vi "Log Data to File.vi"(8 "error in":errorcluster, 10 "Log Data":string[](array[string])) -> (0 "error out":errorcluster)   [LabVIEW 2019]
doc: "This VI writes data to Spreadsheet. Data is logged into Application Directory in CSV format."
uses:
  <vilib>/Utility/file.llb/Write Delimited Spreadsheet (string).vi
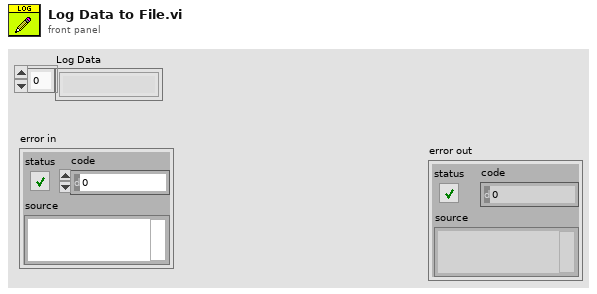
[diagram p1: front panel]
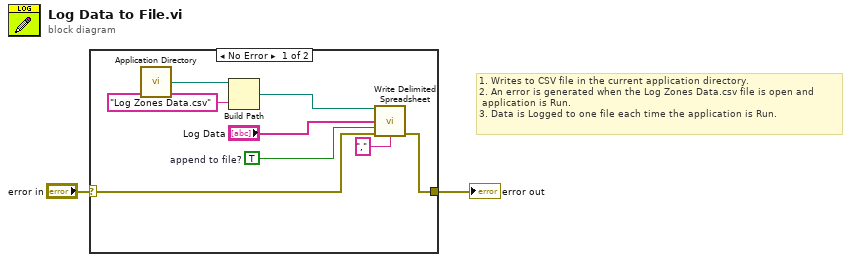
[diagram p0: block diagram]
diagram:
  # "1. Writes to CSV file in the current application directory.\n2. An error is generated when the Log Zones Data.csv file is open and\n application is Run.\n3. Data is Logged to one file each time the application is Run."
  n1 = case shown="No Error" "error in" {
    selector: "error in" -> [w3 w11]
    tunnel: [w4 w11] -> w2
    frame No Error {
      w10 = TRUE  # append to file?
      n2 = call <vilib>:"Application Directory.vi"() -> ("Application Directory"=w7:path)
      n3 = Build Path(base path=w7, name or relative path="Log Zones Data.csv") -> (appended path=w9:path)
      n4 = call-poly <vilib>:"Write Delimited Spreadsheet.vi"("file path (dialog if empty)"=w9, "1D data"="Log Data", "append to file? (new file:F)"=w10, "error in (no error)"=w3, "delimiter (\\t)"="," ("delimiter (\\t)")) -> ("error out"=w4:errorcluster)  [unwired: 9 in, 1 out]
    }
    frame Error {
    }
  }
  "error out" <- w2
